vi "solar_excel Cell Values.vi"(11 "Cells in":string[][](array[string])) -> (3 "Values":string[][](array[string]), 5 "Column Headers (w/o First)":string[](array[string]), 7 "Row Headers (w/o First)":string[](array[string]))   [LabVIEW 2018]
doc: "This removes the Row and Column Headers (first row & first column) and deletes cell 'A1'."
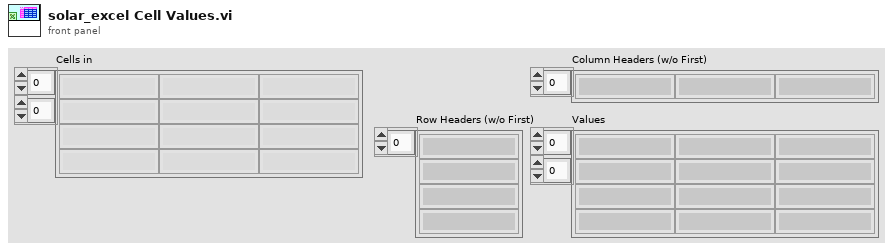
[diagram p1: front panel]
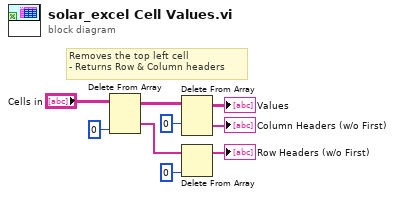
[diagram p0: block diagram]
diagram:
  # "Removes the top left cell\n- Returns Row & Column headers"
  n1 = Delete From Array(array="Cells in", index (col)=0 ("disabled index (col)")) -> (deleted portion=w7:string[], array with subset deleted=w3:string[][])  [unwired: 2 in]
  n2 = Delete From Array(array=w3, index (row)=0 ("index")) -> (deleted portion=→"Column Headers (w/o First)":string[], array with subset deleted=→"Values":string[][])  [unwired: 2 in]
  n3 = Delete From Array(array=w7, index=0) -> (array with subset deleted=→"Row Headers (w/o First)":string[])  [unwired: 1 in, 1 out]
